vi "Read file.vi"(10 "MXN":bool, 11 "Coca in":refnum<class "Coca.lvclass">) -> (2 "Item Names":string[][](array[string]), 3 "path":path)   [LabVIEW 2020, in "Coca.lvlib" / "Coca.lvclass"]
uses:
  Coca.lvclass
  <vilib>/Utility/config.llb/Read Key (String).vi
  <vilib>/Utility/config.llb/NI_LVConfig.lvlib
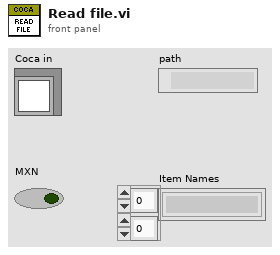
[diagram p1: front panel]
types:
  T1 = typedef "NI_LVConfig.lvlib/Config Data RefNum.ctl" = refnum<k1>
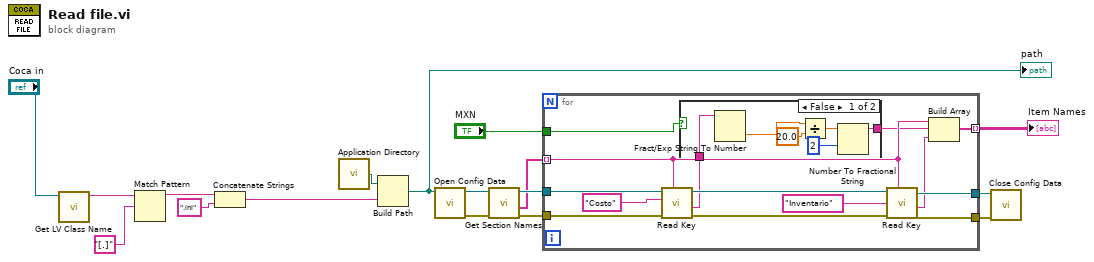
[diagram p0: block diagram]
diagram:
  n1 = call <vilib>:"Get LV Class Name.vi"("object"="Coca in") -> ("class name"=w9:string)  [unwired: 9 in, 1 out]
  n2 = Match Pattern(string=w9, regular expression="[.]") -> (before substring=w16:string)  [unwired: 1 in, 3 out]
  n3 = Concatenate Strings(w16, ".ini" ("string")) -> (w10:string)
  n4 = call <vilib>:"Application Directory.vi"() -> ("Application Directory"=w8:path)
  n5 = Build Path(base path=w8, name or relative path=w10) -> (appended path=w12:path)
  "path" <- w12
  n6 = call <vilib>:"Open Config Data.vi"("configuration file path"=w12) -> ("error out"=w5:errorcluster, "refnum"=w13:T1)  [unwired: 8 in, 1 out]
  n7 = call <vilib>:"Get Section Names.vi"("error in (no error)"=w5, "refnum"=w13) -> ("error out"=w4:errorcluster, "section names"=w3:string[], "refnum out"=w6:T1)  [unwired: 7 in]
  n8 = for {
    tunnel: w4 -> [w31]
    tunnel: w6 -> [w28]
    tunnel: [w27] -> w14
    tunnel: [w26] -> w15
    tunnel: w3 -> [w23] mode=indexing
    tunnel: [w21] -> w2 mode=indexing
    tunnel: "MXN" -> [w18]
    n9 = call-poly <vilib>:"Read Key.vi"("section"=w23, "error in (no error)"=w31, "key"="Costo" ("section"), "refnum"=w28) -> ("error out"=w30:errorcluster, "value"=w20:string, "refnum out"=w29:T1)  [unwired: 4 in, 1 out]
    n10 = case shown="False" w18 {
      tunnel: w20 -> [w35 w38]
      tunnel: [w33 w38] -> w19
      frame False {
        n11 = Fract/Exp String To Number(string=w35) -> (number=w36:dbl)  [unwired: 3 in, 1 out]
        n12 = Divide(x=w36, y=20.0) -> (x/y=w34:dbl)
        n13 = Number To Fractional String(number=w34, precision (6)=i16 2) -> (F-format string=w33:string)  [unwired: 2 in]
      }
      frame True {
      }
    }
    n14 = call-poly <vilib>:"Read Key.vi"("section"=w23, "error in (no error)"=w30, "key"="Inventario" ("section"), "refnum"=w29) -> ("error out"=w27:errorcluster, "value"=w22:string, "refnum out"=w26:T1)  [unwired: 4 in, 1 out]
    n15 = Build Array(w23, w19, w22) -> (w21:string[])
  }
  "Item Names" <- w2
  n16 = call <vilib>:"Close Config Data.vi"("error in (no error)"=w14, "refnum"=w15) -> ()  [unwired: 8 in, 2 out]
